vi "CryptoNight-SingleRound-Top-Level.vi"(10 "state (c)":u32[](array[numeric]) format="%.0x", 11 "key (a)":u64[](array[numeric]) format="%.0x") -> (3 "state out (c)":u32[](array[numeric]) format="%.0x")   [LabVIEW 2017]
uses:
  xtime.vi
panel:
  out "MATCH":bool
  out "expected\nstate out (c)":u32[](array[numeric]) format="%.0x"
  out "ADD_KEY":u8[](array[numeric]) format="%.0x"
  out "MIX_COLUMNS":u8[](array[numeric]) format="%.0x"
  out "SHIFT_ROWS":u8[](array[numeric]) format="%.0x"
  out "SUB_BYTES":u8[](array[numeric]) format="%.0x"
  # "SHIFT_ROWS\n0043ad66 1d829e4f\n39b8a31f ea3a1509"
  # "SUB_BYTES\n631a9533 a4130b84\n126c0ac0 87805901"
  # "MIX_COLUMNS\n4ec01d4c e91b36fc\n5a1431cb d676b649"
  # "ADD_KEY\n8f0a14e7 cbadf9f5 \n66e5e47e 34a38893"
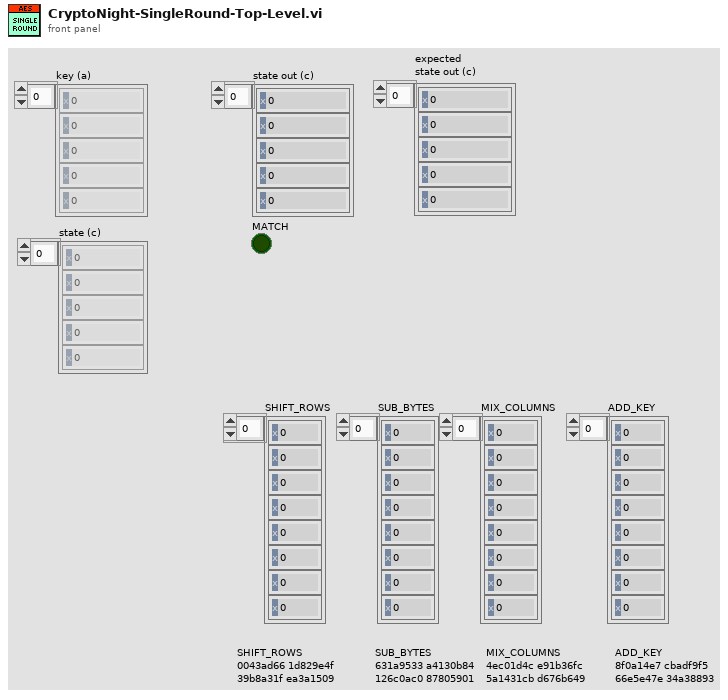
[diagram p1: front panel]
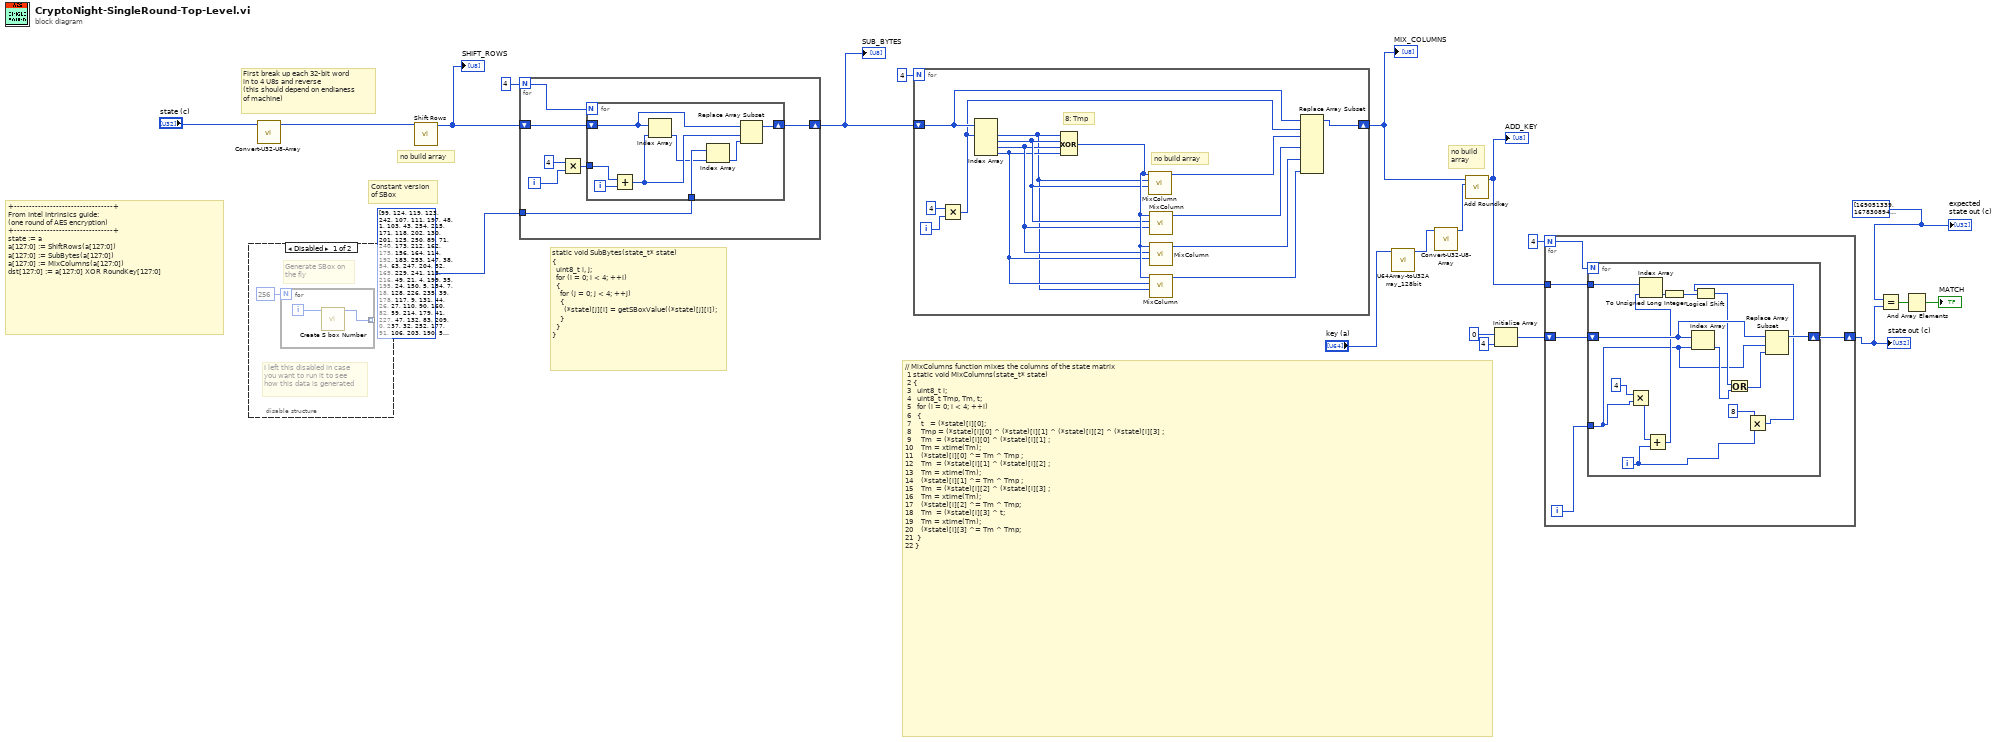
[diagram p0: block diagram]
diagram:
  w3 = u32[] [169051339, 1678308948, 1571005530, 2110178431] ("expected\nstate out (c)")
  # "no build\narray"
  # "no build array"
  # "Constant version\nof SBox"
  # "// MixColumns function mixes the columns of the state matrix\n 1 static void MixColumns(state_t* state)\n 2 {\n 3   uint8_t i;\n 4   uint8_t Tmp, Tm, t;\n 5   for (i = 0; i < 4; ++i)\n 6   {  \n 7     t   = (*state)[i][0]; \n 8     Tmp = (*state)[i][0] ^ (*state)[i][1] ^ (*state)[i][2] ^ (*state)[i][3] ;\n 9     Tm  = (*state)[i][0] ^ (*state)[i][1] ;\n10    Tm = xtime(Tm);  \n11    (*state)[i][0] ^= Tm ^ Tmp ;\n12    Tm  = (*state)[i][1] ^ (*state)[i][2] ; \n13    Tm = xtime(Tm);  \n14    (*state)[i][1] ^= Tm ^ Tmp ;\n15    Tm  = (*state)[i][2] ^ (*state)[i][3] ;\n16    Tm = xtime(Tm);\n17    (*state)[i][2] ^= Tm ^ Tmp;\n18    Tm  = (*state)[i][3] ^ t;\n19    Tm = xtime(Tm);\n20    (*state)[i][3] ^= Tm ^ Tmp;\n21  }\n22 }"
  # "static void SubBytes(state_t* state)\n{\n  uint8_t i, j;\n  for (i = 0; i < 4; ++i)\n  {\n    for (j = 0; j < 4; ++j)\n    {\n      (*state)[j][i] = getSBoxValue((*state)[j][i]);\n    }\n  }\n}"
  # "First break up each 32-bit word\nin to 4 U8s and reverse\n(this should depend on endianess\nof machine)"
  # "+---------------------------------+\nFrom Intel Intrinsics guide:\n(one round of AES encryption)\n+---------------------------------+\nstate := a\na[127:0] := ShiftRows(a[127:0])\na[127:0] := SubBytes(a[127:0])\na[127:0] := MixColumns(a[127:0])\ndst[127:0] := a[127:0] XOR RoundKey[127:0]"
  n1 = disable-structure shown="Disabled" {
    frame Disabled {
      # "I left this disabled in case\nyou want to run it to see\nhow this data is generated"
      # "Generate SBox on\nthe fly"
      n2 = for {
        N: 256 -> [_]
        tunnel: [w22] -> _ mode=indexing
        i -> [w23]
        n3 = call "Create S box Number.vi"("Index"=w23) -> ("S-Box"=w22:u8)  [unwired: 10 in]
      }
    }
    frame Enabled {
    }
  }
  n4 = call "Convert-U32-U8-Array.vi"("state"="state (c)") -> ("Array"=w20:u8[])  [unwired: 10 in]
  n5 = call "Shift Rows.vi"("Data In"=w20) -> ("Data Out"=w18:u8[])  [unwired: 10 in]
  "SHIFT_ROWS" <- w18
  n6 = for {
    N: 4 -> [w30]
    shift-right: [w27] -> w16
    shift-left: w18 -> [w29]
    tunnel: u8[] [99, 124, 119, 123, 242, 107, 111, 197, 48, 1, 103, 43, 254, 215, 171, 118, 202, 130, 201, 125, 250, 89, 71, 240, 173, 212, 162, 175, 156, 164, 114, 192, 183, 253, 147, 38, 54, 63, 247, 204, 52, 165, 229, 241, 113, 216, 49, 21, 4, 199, 35, 195, 24, 150, 5, 154, 7, 18, 128, 226, 235, 39, 178, 117, 9, 131, 44, 26, 27, 110, 90, 160, 82, 59, 214, 179, 41, 227, 47, 132, 83, 209, 0, 237, 32, 252, 177, 91, 106, 203, 190, 57, 74, 76, 88, 207, 208, 239, 170, 251, 67, 77, 51, 133, 69, 249, 2, 127, 80, 60, 159, 168, 81, 163, 64, 143, 146, 157, 56, 245, 188, 182, 218, 33, 16, 255, 243, 210, 205, 12, 19, 236, 95, 151, 68, 23, 196, 167, 126, 61, 100, 93, 25, 115, 96, 129, 79, 220, 34, 42, 144, 136, 70, 238, 184, 20, 222, 94, 11, 219, 224, 50, 58, 10, 73, 6, 36, 92, 194, 211, 172, 98, 145, 149, 228, 121, 231, 200, 55, 109, 141, 213, 78, 169, 108, 86, 244, 234, 101, 122, 174, 8, 186, 120, 37, 46, 28, 166, 180, 198, 232, 221, 116, 31, 75, 189, 139, 138, 112, 62, 181, 102, 72, 3, 246, 14, 97, 53, 87, 185, 134, 193, 29, 158, 225, 248, 152, 17, 105, 217, 142, 148, 155, 30, 135, 233, 206, 85, 40, 223, 140, 161, 137, 13, 191, 230, 66, 104, 65, 153, 45, 15, 176, 84, 187, 22] ("Array") -> [w28]
    i -> [w26]
    n7 = Multiply(x=4, y=w26) -> (x*y=w24:i32)
    n8 = for {
      N: w30 -> [_]
      tunnel: w24 -> [w38]
      shift-right: [w31] -> w27
      shift-left: w29 -> [w36]
      tunnel: w28 -> [w34]
      i -> [w37]
      n9 = Add(x=w38, y=w37) -> (x+y=w35:i32)
      n10 = Index Array(array=w36, index=w35) -> (element=w33:u8)
      n11 = Index Array(array=w34, index=w33) -> (element=w32:u8)
      n12 = Replace Array Subset(array=w36, new element=w32, index=w35) -> (w31:u8[])
    }
  }
  "SUB_BYTES" <- w16
  n13 = for {
    N: 4 -> [_]
    shift-right: [w39] -> w15
    shift-left: w16 -> [w50]
    i -> [w51]
    # "no build array"
    # "8: Tmp"
    n14 = Multiply(x=4, y=w51) -> (x*y=w49:i32)
    n15 = Index Array(array=w50, index #1=w49) -> (element #1=w40:u8, element #2=w43:u8, element #3=w42:u8, element #4=w41:u8)  [unwired: 3 in]
    n16 = Compound Arithmetic op=XOR(w40, w43, w42, w41) -> (w44:u8)
    n17 = call "MixColumn.vi"("state[i][y]"=w43, "state[i][x]"=w40, "Tmp"=w44) -> ("state[i][x]"=w48:u8)  [unwired: 8 in]
    n18 = call "MixColumn.vi"("state[i][y]"=w42, "state[i][x]"=w43, "Tmp"=w44) -> ("state[i][x]"=w47:u8)  [unwired: 8 in]
    n19 = call "MixColumn.vi"("state[i][y]"=w41, "state[i][x]"=w42, "Tmp"=w44) -> ("state[i][x]"=w46:u8)  [unwired: 8 in]
    n20 = call "MixColumn.vi"("state[i][y]"=w40, "state[i][x]"=w41, "Tmp"=w44) -> ("state[i][x]"=w45:u8)  [unwired: 8 in]
    n21 = Replace Array Subset(array=w50, new element #1=w48, index #1=w49, new element #2=w47, new element #3=w46, new element #4=w45) -> (w39:u8[])  [unwired: 3 in]
  }
  "MIX_COLUMNS" <- w15
  n22 = call "U64Array-toU32Array_128bit.vi"("2 x U64"="key (a)") -> ("4 x U32"=w6:u32[])  [unwired: 10 in]
  n23 = call "Convert-U32-U8-Array.vi"("state"=w6) -> ("Array"=w14:u8[])  [unwired: 10 in]
  n24 = call "Add Roundkey.vi"("Roundkey In"=w14, "Data In"=w15) -> ("Array Out"=w12:u8[])  [unwired: 9 in]
  "ADD_KEY" <- w12
  n25 = Initialize Array(u32 0 ("element"), 4 ("dimension size")) -> (w9:u32[])
  n26 = for {
    N: 4 -> [w57]
    tunnel: w12 -> [w55]
    shift-right: [w54] -> w4
    shift-left: w9 -> [w56]
    i -> [w53]
    n27 = for {
      N: w57 -> [_]
      tunnel: w53 -> [w59]
      shift-right: [w67] -> w54
      shift-left: w56 -> [w72]
      tunnel: w55 -> [w71]
      i -> [w64]
      n28 = Multiply(x=4, y=w59) -> (x*y=w58:i32)
      n29 = Add(x=w58, y=w64) -> (x+y=w70:i32)
      n30 = Index Array(array=w71, index=w70) -> (element=w66:u8)
      n31 = To Unsigned Long Integer(number=w66) -> (unsigned 32bit integer=w61:u32)
      n32 = Index Array(array=w72, index=w59) -> (element=w69:u32)
      n33 = Multiply(x=8, y=w64) -> (x*y=w62:i32)
      n34 = Logical Shift(y=w62, x=w61) -> (x << y=w65:u32)
      n35 = Or(x=w65, y=w69) -> (x .or. y?=w68:u32)
      n36 = Replace Array Subset(array=w72, new element=w68, index=w59) -> (w67:u32[])
    }
  }
  "state out (c)" <- w4
  n37 = Equal?(x=w3, y=w4) -> (x = y?=w2:bool[])
  n38 = And Array Elements(Boolean array=w2) -> (logical AND=→"MATCH":bool)
  "expected\nstate out (c)" <- w3
